vi "half adder_0.vi"(10 "switch 2":bool, 11 "switch 1":bool) -> (2 "sum":bool, 3 "carry":bool)   [LabVIEW 2015]
panel:
  in  "Tab Control":enum32{"Page 1", "Page 2"}(tab)
  # "Pardeeop Kumar"
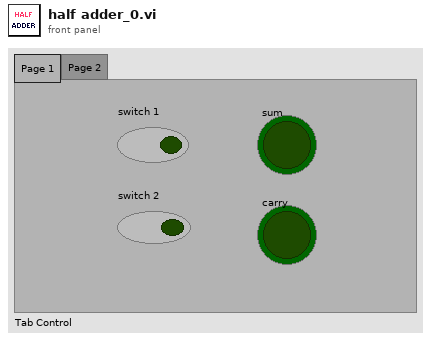
[diagram p1: front panel]
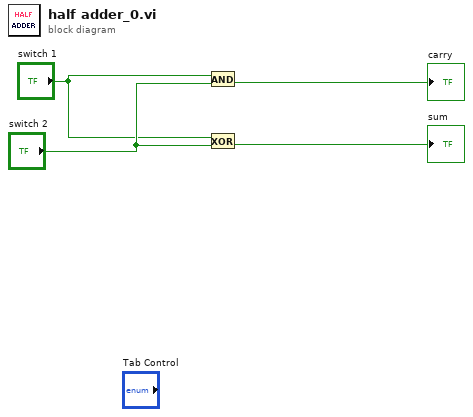
[diagram p0: block diagram]
diagram:
  n1 = And(x="switch 1", y="switch 2") -> (x .and. y?=→"carry":bool)
  n2 = Exclusive Or(1:"switch 2", 2:"switch 1") -> (0:→"sum":bool)
